vi "MainScreen.vi"() -> ()   [LabVIEW 2020]
uses:
  <vilib>/event_ctls.llb/eventsource.ctl
  <vilib>/DAQmx/write.llb/DAQmx Write (Digital Bool 1Line 1Point).vi
  <vilib>/DAQmx/read.llb/DAQmx Read (Analog 1D DBL NChan 1Samp).vi
  <vilib>/DAQmx/create/channels.llb/DAQmx Create Channel (DO-Digital Output).vi
  <vilib>/DAQmx/miscellaneous.llb/DAQmx Fill In Error Info.vi
  <vilib>/Utility/file.llb/Write Delimited Spreadsheet (string).vi
  <vilib>/Utility/file.llb/Write Delimited Spreadsheet (DBL).vi
  <vilib>/ErrorRing/Error Ring.xnode
  <vilib>/vision/driver/NI_Vision_Acquisition_Software.lvlib
panel:
  in  "New Experiment":bool
  in  "Laser On":bool
  in  "physical channels 2":tag="cDAQ1Mod5/ai1,cDAQ1Mod5/ai2"
  out "Saving Data":bool
  out "System Time":dbl
  in  "Sample Rate":dbl=90.0
  out "error out 2":errorcluster
  out "Image 2":T1(plugin-control)
  out "Image":T1(plugin-control)
  out "error out":errorcluster
  out "Clock":dbl[](graph)
  out "T.C 2":dbl[](graph)
  out "T.C 3":dbl[](graph)
  out "T.C 4":dbl[](graph)
  out "T.C 5":dbl[](graph)
  out "T.C 6":dbl[](graph)
  out "T.C 7":dbl[](graph)
  out "Rear Diode":dbl[](graph)
  out "Front Diode":dbl[](graph)
  out "T.C 1":dbl[](graph)
  out "T.C 8":dbl[](graph)
  in  "stop":bool
  in  "TC channel":tag="cDAQ1Mod4/ai0,cDAQ1Mod4/ai1,cDAQ1Mod4/ai2,cDAQ1Mod4/ai3,cDAQ1Mod4/ai4,cDAQ1Mod4/ai5,cDAQ1Mod4/ai6,cDAQ1Mod4/ai7"
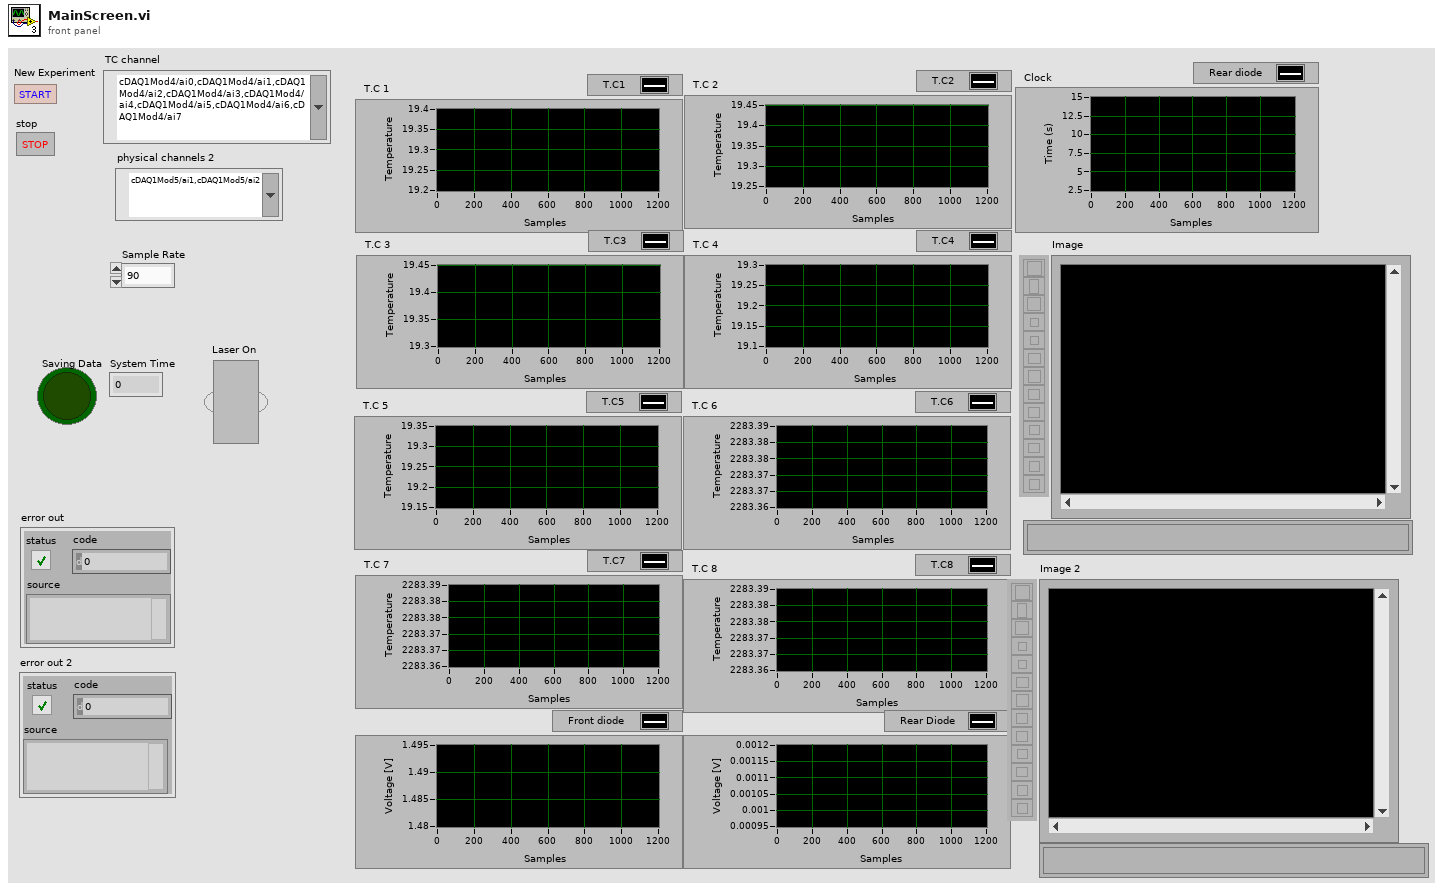
[diagram p1: front panel]
types:
  T1 = typedef "IMAQ Image.ctl" = refnum<image>
  T2 = typedef "eventsource.ctl" = u32
  T3 = typedef "IMAQ AVI2 Refnum.ctl" = refnum<k20>
  T4 = typedef "IMAQdx.ctl" = refnum<k21>
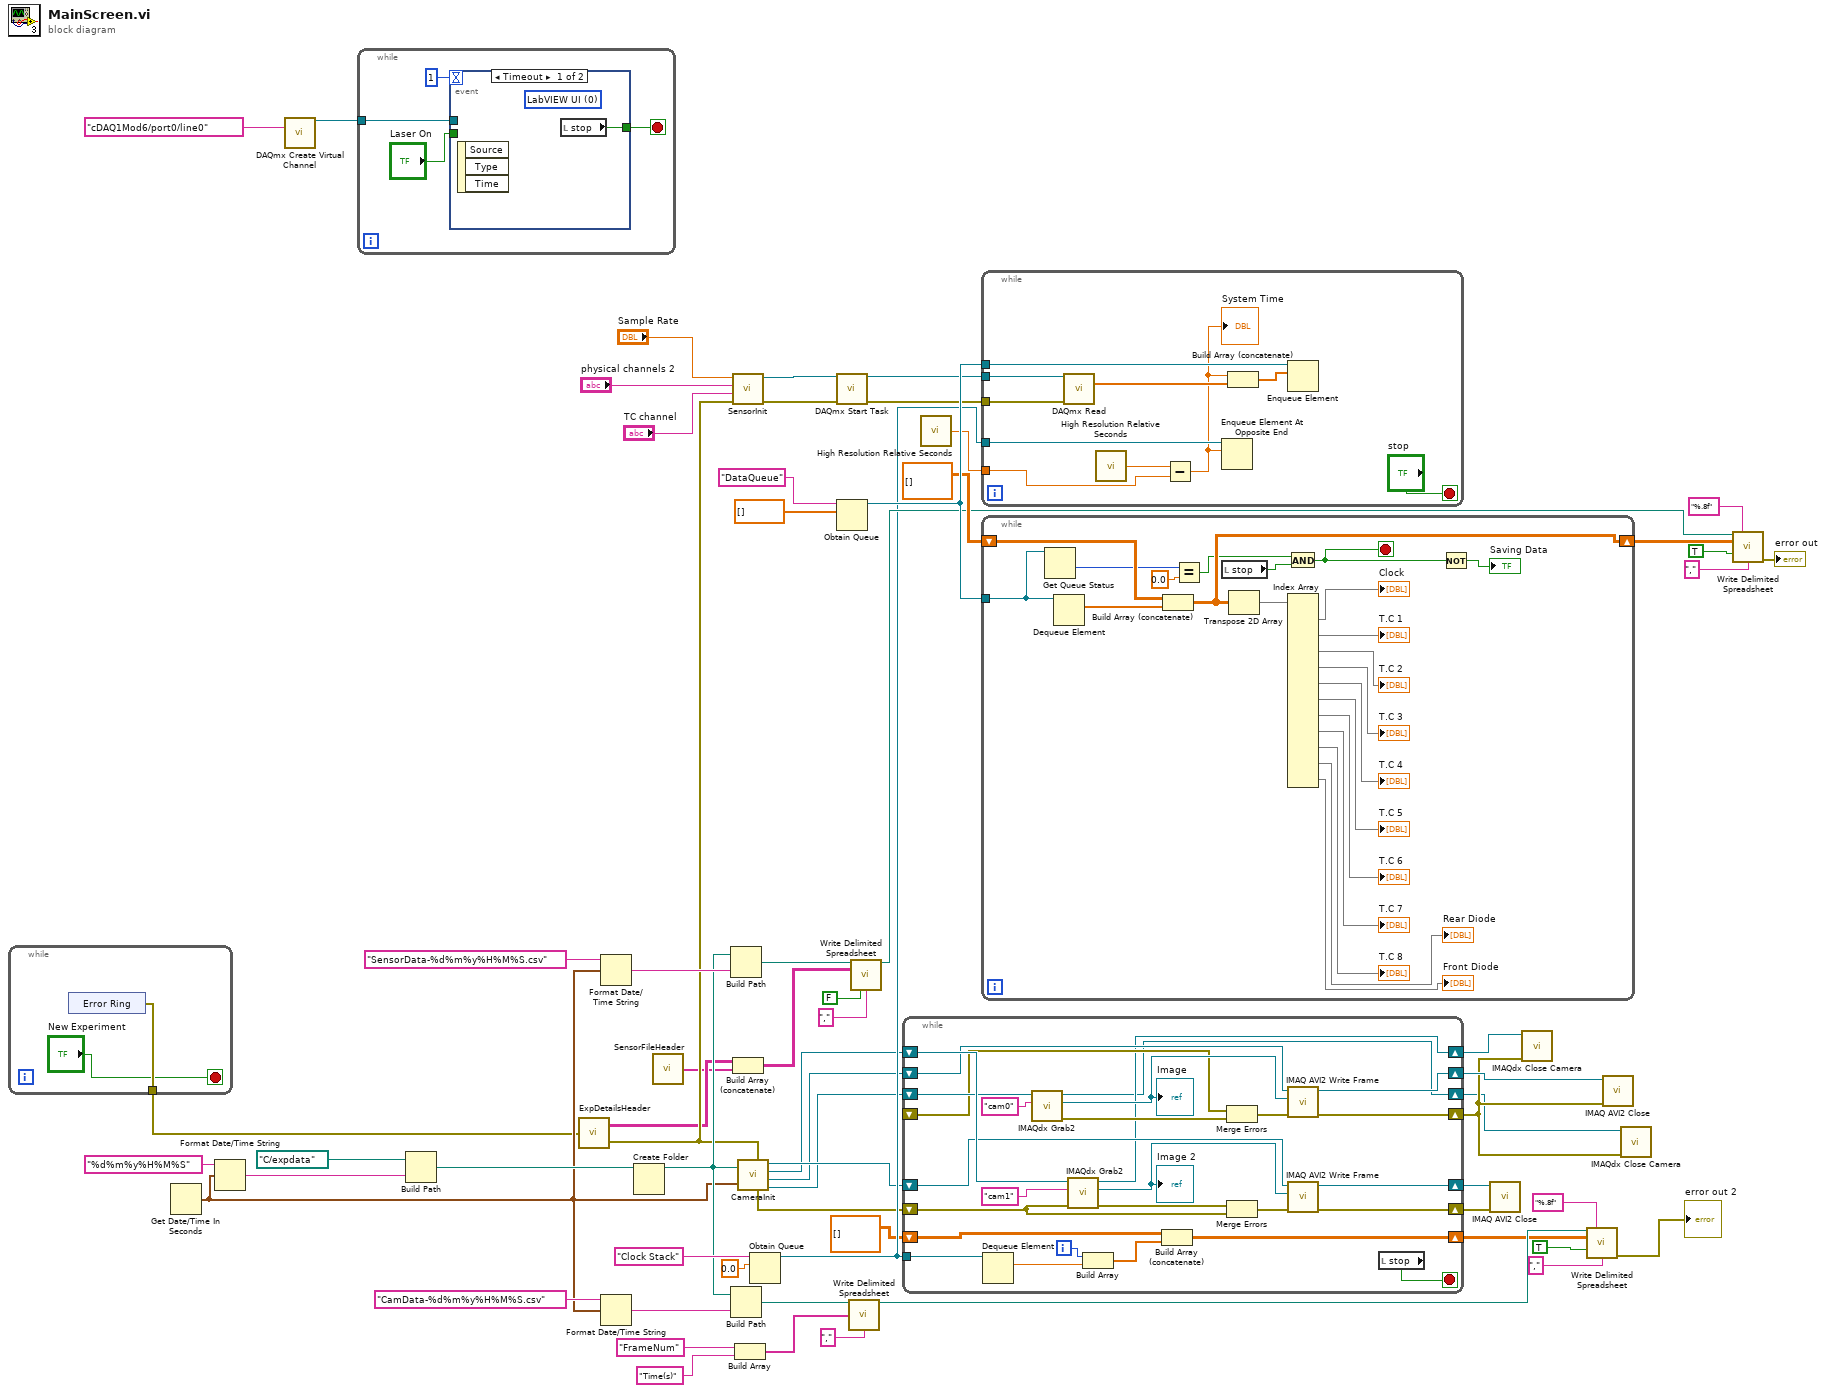
[diagram p0: block diagram]
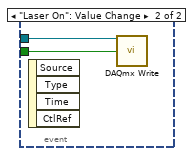
[diagram p2: hidden frame]
diagram:
  n1 = while {
    tunnel: [w66] -> w1
    stop <- "New Experiment" stop-if-true
    n2 = xnode "Error Ring"() -> ("error out"=w66:errorcluster)
  }
  n3 = Get Date/Time In Seconds() -> (seconds since 1Jan1904=w9:timestamp)
  n4 = Format Date/Time String(time format string (%c)="%d%m%y%H%M%S", seconds (now)=w9) -> (date/time string=w52:string)  [unwired: 1 in]
  n5 = call-poly <vilib>:"DAQmx Create Virtual Channel.vi"("lines"=tag "cDAQ1Mod6/port0/line0") -> ("task out"=w7:refnum<k21>)  [unwired: 13 in, 1 out]
  n6 = while {
    tunnel: w7 -> [w71]
    stop <- w68 stop-if-true
    n7 = event shown="[0] Timeout" {
      selector: _ -> [_ _]
      dyn-events: _ -> [_ _]
      timeout: 1 -> [_ _]
      tunnel: w71 -> [_ w74]
      tunnel: "Laser On" -> [_ w73]
      tunnel: [w72 _] -> w68
      event Timeout {
        (unwired) T2 0 items=["LabVIEW UI"=0, "ActiveX"=1, "User Event"=25] ("Source")
        n8 = event-data() -> ()  [unwired: 1 in, 3 out]
        n9 = local read "stop"() -> (w72:bool)
      }
      event "Laser On": Value Change {
        n10 = event-data() -> ()  [unwired: 1 in, 4 out]
        n11 = call-poly <vilib>:"DAQmx Write.vi"("task/channels in"=w74, "data"=w73) -> ()  [unwired: 11 in, 3 out]
      }
    }
  }
  n12 = Build Path(base path=path "C:/expdata", name or relative path=w52) -> (appended path=w51:path)
  n13 = call "ExpDetailsHeader.vi"("error in (no error)"=w1) -> ("appended array"=w3:string[][], "error out"=w5:errorcluster)
  n14 = Format Date/Time String(time format string (%c)="SensorData-%d%m%y%H%M%S.csv", seconds (now)=w9) -> (date/time string=w49:string)  [unwired: 1 in]
  n15 = Format Date/Time String(time format string (%c)="CamData-%d%m%y%H%M%S.csv", seconds (now)=w9) -> (date/time string=w31:string)  [unwired: 1 in]
  n16 = Create Folder(path (use dialog)=w51) -> (created path=w10:path)  [unwired: 2 in, 2 out]
  n17 = call "SensorFileHeader.vi"() -> ("Header\nOut"=w2:string[])
  n18 = Build Path(base path=w10, name or relative path=w49) -> (appended path=w48:path)
  n19 = Build Path(base path=w10, name or relative path=w31) -> (appended path=w30:path)
  n20 = call "SensorInit.vi"("error in (no error)"=w5, "TC channel"="TC channel", "physical channels in"="physical channels 2", "Sample Rate"="Sample Rate") -> ("error out"=w57:errorcluster, "Task out"=w59:refnum<k21>)  [unwired: 6 in]
  n21 = Build Array (concatenate)(w3, w2) -> (w4:string[][])
  n22 = Build Array("FrameNum", "Time(s)") -> (w26:string[])
  n23 = call "CameraInit.vi"("folder path"=w10, "start time"=w9, "error in (no error)"=w5) -> ("error out"=w6:errorcluster, "Color AVI out"=w14:T3, "Color session out"=w13:T4, "BW AVI out"=w12:T3, "BW Session Out"=w11:T4)
  n24 = Obtain Queue(name (unnamed)="Clock Stack", element data type=0.0) -> (queue out=w33:refnum<queue>)  [unwired: 3 in, 2 out]
  n25 = call <vilib>:"DAQmx Start Task.vi"("task/channels in"=w59, "error in"=w57) -> ("task out"=w58:refnum<k21>, "error out"=w56:errorcluster)  [unwired: 12 in]
  n26 = Obtain Queue(name (unnamed)="DataQueue", element data type=dbl[] []) -> (queue out=w64:refnum<queue>)  [unwired: 3 in, 2 out]
  n27 = call-poly <vilib>:"Write Delimited Spreadsheet.vi"("file path (dialog if empty)"=w30, "1D data"=w26, "delimiter (\\t)"="," ("delimiter (\\t)")) -> ("new file path (Not A Path if cancelled)"=w22:path)  [unwired: 11 in, 1 out]
  n28 = call-poly <vilib>:"Write Delimited Spreadsheet.vi"("file path (dialog if empty)"=w48, "2D data"=w4, "transpose? (no:F)"=FALSE, "delimiter (\\t)"="," ("delimiter (\\t)")) -> ("new file path (Not A Path if cancelled)"=w42:path)  [unwired: 10 in, 1 out]
  n29 = while {
    shift-right: [w86] -> w36
    shift-left: w13 -> [w99]
    shift-right: [w88] -> w38
    shift-left: w6 -> [w75]
    shift-right: [w90] -> w40
    shift-left: w14 -> [w98]
    shift-right: [w85] -> w35
    shift-left: w11 -> [w95]
    shift-right: [w89] -> w39
    shift-left: w12 -> [w94]
    shift-right: [w87] -> w37
    shift-left: _ -> [w92]
    tunnel: w33 -> [w84]
    shift-right: [w81] -> w21
    shift-left: dbl[][] [] -> [w82]
    i -> [w79]
    stop <- w80 stop-if-true
    n30 = Dequeue Element(queue=w84) -> (element=w78:dbl)  [unwired: 2 in, 3 out]
    n31 = call <vilib>:"IMAQdx Grab2.vi"("Image In"="cam0" ("Image Name"), "Session In"=w95) -> ("error out"=w93:errorcluster, "Image Out"=w101:T1, "Session Out"=w85:T4)  [unwired: 6 in, 1 out]
    "Image" <- w101
    n32 = call <vilib>:"IMAQdx Grab2.vi"("error in"=w75, "Image In"="cam1" ("Image Name"), "Session In"=w99) -> ("error out"=w96:errorcluster, "Image Out"=w100:T1, "Session Out"=w86:T4)  [unwired: 5 in, 1 out]
    "Image 2" <- w100
    n33 = Build Array(w79, w78) -> (w83:dbl[])
    n34 = Build Array (concatenate)(w82, w83) -> (w81:dbl[][])
    n35 = Merge Errors(w92, w93) -> (w91:errorcluster)
    n36 = Merge Errors(w96, w75) -> (w97:errorcluster)
    n37 = call "IMAQ AVI2 Write Frame"("error in (no error)"=w91, "Image"=w101, "AVI Refnum"=w94) -> ("error out"=w87:errorcluster, "AVI Refnum (duplicate)"=w89:T3)  [unwired: 6 in, 1 out]
    n38 = call "IMAQ AVI2 Write Frame"("error in (no error)"=w97, "Image"=w100, "AVI Refnum"=w98) -> ("error out"=w88:errorcluster, "AVI Refnum (duplicate)"=w90:T3)  [unwired: 6 in, 1 out]
    n39 = local read "stop"() -> (w80:bool)
  }
  n40 = call <vilib>:"High Resolution Relative Seconds.vi"() -> ("relative seconds"=w60:dbl)
  n41 = while {
    tunnel: w64 -> [w111]
    tunnel: w58 -> [w110]
    tunnel: w56 -> [w109]
    tunnel: w60 -> [w108]
    tunnel: w33 -> [w103]
    stop <- "stop" stop-if-true
    n42 = call-poly <vilib>:"DAQmx Read.vi"("task/channels in"=w110, "error in"=w109) -> ("data"=w106:dbl[])  [unwired: 11 in, 2 out]
    n43 = call <vilib>:"High Resolution Relative Seconds.vi"() -> ("relative seconds"=w107:dbl)
    n44 = Subtract(x=w107, y=w108) -> (x-y=w102:dbl)
    "System Time" <- w102
    n45 = Enqueue Element At Opposite End(queue=w103, element=w102) -> ()  [unwired: 2 in, 3 out]
    n46 = Build Array (concatenate)(w102, w106) -> (w105:dbl[])
    n47 = Enqueue Element(queue=w111, element=w105) -> ()  [unwired: 2 in, 3 out]
  }
  n48 = while {
    tunnel: w64 -> [w116]
    shift-right: [w120] -> w43
    shift-left: dbl[][] [] -> [w133]
    stop <- w113 stop-if-true
    n49 = Get Queue Status(queue=w116) -> (# pending insert=w115:i32)  [unwired: 2 in, 7 out]
    n50 = Dequeue Element(queue=w116) -> (element=w132:dbl[])  [unwired: 2 in, 3 out]
    n51 = Build Array (concatenate)(w133, w132) -> (w120:dbl[][])
    n52 = Equal?(x=w115, y=0.0) -> (x = y?=w118:bool)
    n53 = local read "stop"() -> (w114:bool)
    n54 = Transpose 2D Array(2D array=w120) -> (transposed array=w119:dbl[][])
    n55 = And(x=w118, y=w114) -> (x .and. y?=w113:bool)
    n56 = Index Array(array=w119) -> (element #1=→"Clock":dbl[], element #2=→"T.C 1":dbl[], element #3=→"T.C 2":dbl[], element #4=→"T.C 3":dbl[], element #5=→"T.C 4":dbl[], element #6=→"T.C 5":dbl[], element #7=→"T.C 6":dbl[], element #8=→"T.C 7":dbl[], element #9=→"T.C 8":dbl[], element #10=→"Rear Diode":dbl[], element #11=→"Front Diode":dbl[])  [unwired: 22 in]
    n57 = Not(x=w113) -> (.not. x?=→"Saving Data":bool)
  }
  n58 = call "IMAQ AVI2 Close"("error in (no error)"=w38, "AVI Refnum"=w40) -> ()  [unwired: 9 in, 1 out]
  n59 = call <vilib>:"IMAQdx Close Camera.vi"("error in"=w37, "Session In"=w36) -> ()  [unwired: 9 in, 1 out]
  n60 = call-poly <vilib>:"Write Delimited Spreadsheet.vi"("file path (dialog if empty)"=w22, "format (%.3f)"="%.8f", "2D data"=w21, "append to file? (new file:F)"=TRUE, "delimiter (\\t)"="," ("delimiter (\\t)")) -> ("error out"=→"error out 2":errorcluster)  [unwired: 9 in, 1 out]
  n61 = call "IMAQ AVI2 Close"("error in (no error)"=w37, "AVI Refnum"=w39) -> ()  [unwired: 9 in, 1 out]
  n62 = call <vilib>:"IMAQdx Close Camera.vi"("error in"=w37, "Session In"=w35) -> ()  [unwired: 9 in, 1 out]
  n63 = call-poly <vilib>:"Write Delimited Spreadsheet.vi"("file path (dialog if empty)"=w42, "format (%.3f)"="%.8f", "2D data"=w43, "append to file? (new file:F)"=TRUE, "delimiter (\\t)"="," ("delimiter (\\t)")) -> ("error out"=→"error out":errorcluster)  [unwired: 9 in, 1 out]
